vi "appendName.vi"(8 "error in (no error)":errorcluster, 10 "Array String":string[](array[string]), 11 "Category in":refnum<class "Category.lvclass">) -> (0 "error out":errorcluster, 2 "Array String Out":string[](array[string]), 3 "Category out":refnum<class "Category.lvclass">)   [LabVIEW 2018]
uses:
  Category.lvclass
  C:/GitRepos/Filthy-Lucre-Budgetizer/source/support/classes/UserEditableAmount/UserEditableAmount.lvclass
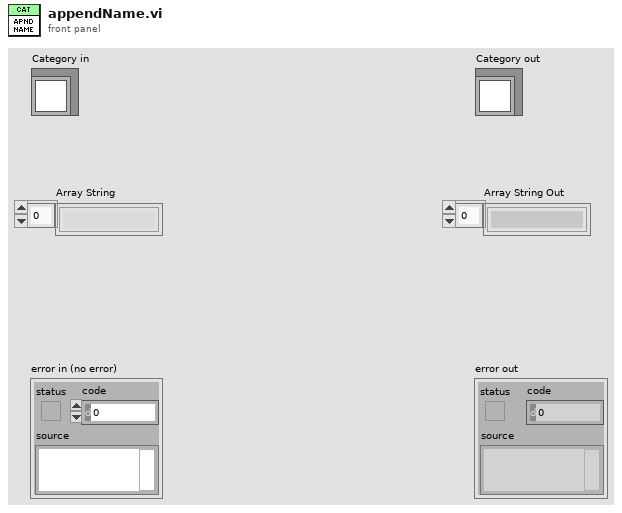
[diagram p1: front panel]
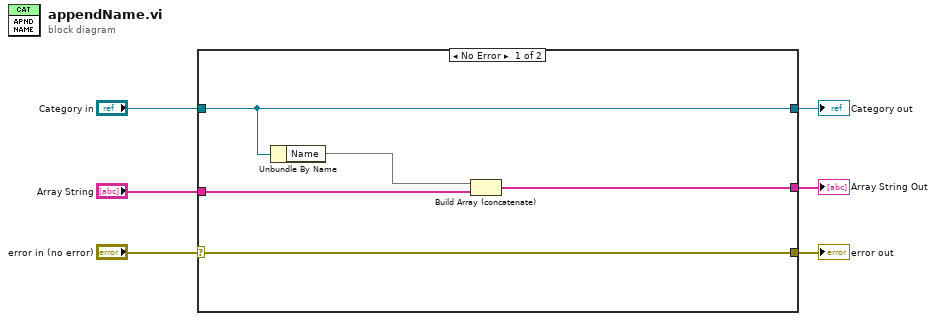
[diagram p0: block diagram]
diagram:
  n1 = case shown="No Error" "error in (no error)" {
    selector: "error in (no error)" -> [w11 w13]
    tunnel: [w11 w13] -> w5
    tunnel: [w10 w12] -> w3
    tunnel: "Category in" -> [w10 w12]
    tunnel: "Array String" -> [w8 _]
    tunnel: [w7 _] -> w1
    frame No Error {
      n2 = Unbundle By Name(w10) -> ("Name"=w9)
      n3 = Build Array (concatenate)(w9, w8) -> (w7:string[])
    }
    frame Error {
    }
  }
  "error out" <- w5
  "Category out" <- w3
  "Array String Out" <- w1
